vi "testWegzähler.vi"() -> ()   [LabVIEW 2013]
uses:
  <vilib>/measure/NI_MAPro.lvlib
panel:
  out "Signalverlaufsdiagramm 2":u32(graph)
  out "Signalverlaufsdiagramm":waveform(dbl)(graph)
  in  "Stopp":bool
  out "Numerisch 2":u32
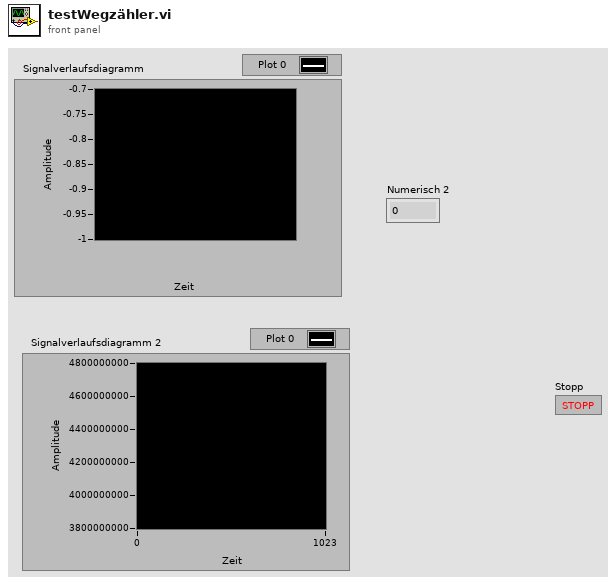
[diagram p1: front panel]
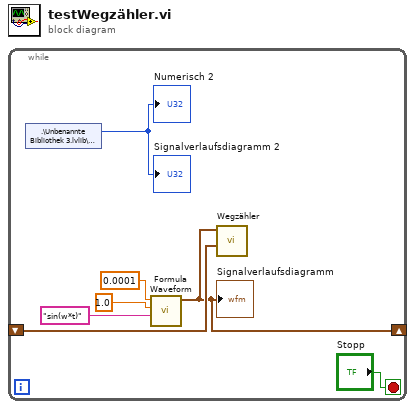
[diagram p0: block diagram]
diagram:
  n1 = while {
    shift-right: [w2] -> _
    shift-left: _ -> [w3]
    stop <- "Stopp" stop-if-true
    n2 = shared-variable ".\\Unbenannte Bibliothek 3.lvlib\\Daten"() -> (→"Numerisch 2" →"Signalverlaufsdiagramm 2":u32)  [unwired: 1 in, 1 out]
    n3 = call <vilib>:"Formula Waveform.vi"("formula"="sin(w*t)", "amplitude"=1.0, "frequency"=0.0001) -> ("signal out"=w2:waveform(dbl))  [unwired: 7 in, 1 out]
    "Signalverlaufsdiagramm" <- w2
    n4 = call "Wegzähler.vi"("letzter Wert"=w3, "aktueller Wert"=w2) -> ()  [unwired: 9 in, 1 out]
  }
